vi "EvaluateVariableValues.vi"(8 "error in (no error)":errorcluster, 11 "VariableManager in":refnum<class "VariableManager.lvclass">) -> (0 "error out":errorcluster, 3 "VariableManager out":refnum<class "VariableManager.lvclass">)   [LabVIEW 2013, in "VariableManager.lvclass"]
doc: "Evaluate variable values and store for future acquisition.\n\nAn error is thrown if a sequence function cannot be evaluated."
uses:
  VariableManager.lvclass
  VariableValue/VariableValue.lvclass
  Variable/Variable.lvclass
  PackedLibraries/LuaEvaluatorAPI.lvlibp/API/t_Caching_Expression_Evaluator_Methods_v4.ctl
  SequenceIndex/SequenceIndex.lvclass
  PackedLibraries/LuaEvaluatorAPI.lvlibp
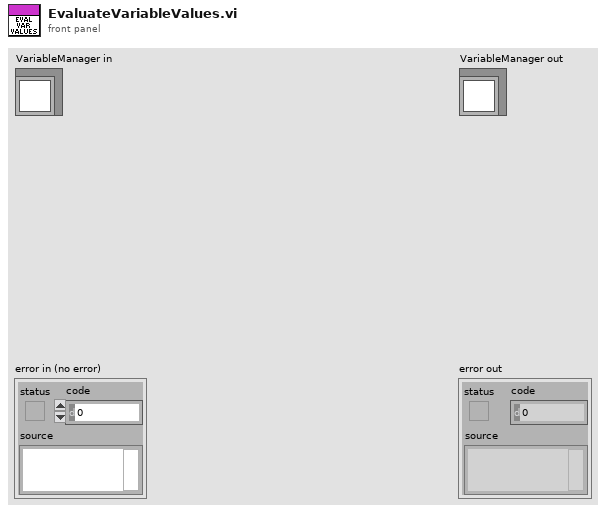
[diagram p1: front panel]
types:
  T1 = typedef "LuaEvaluatorAPI.lvlibp/t_Caching_Expression_Evaluator_Methods_v4.ctl" = enum16{"set", "get", "eval", "eval2", "assign", "execute", "isvalid"}
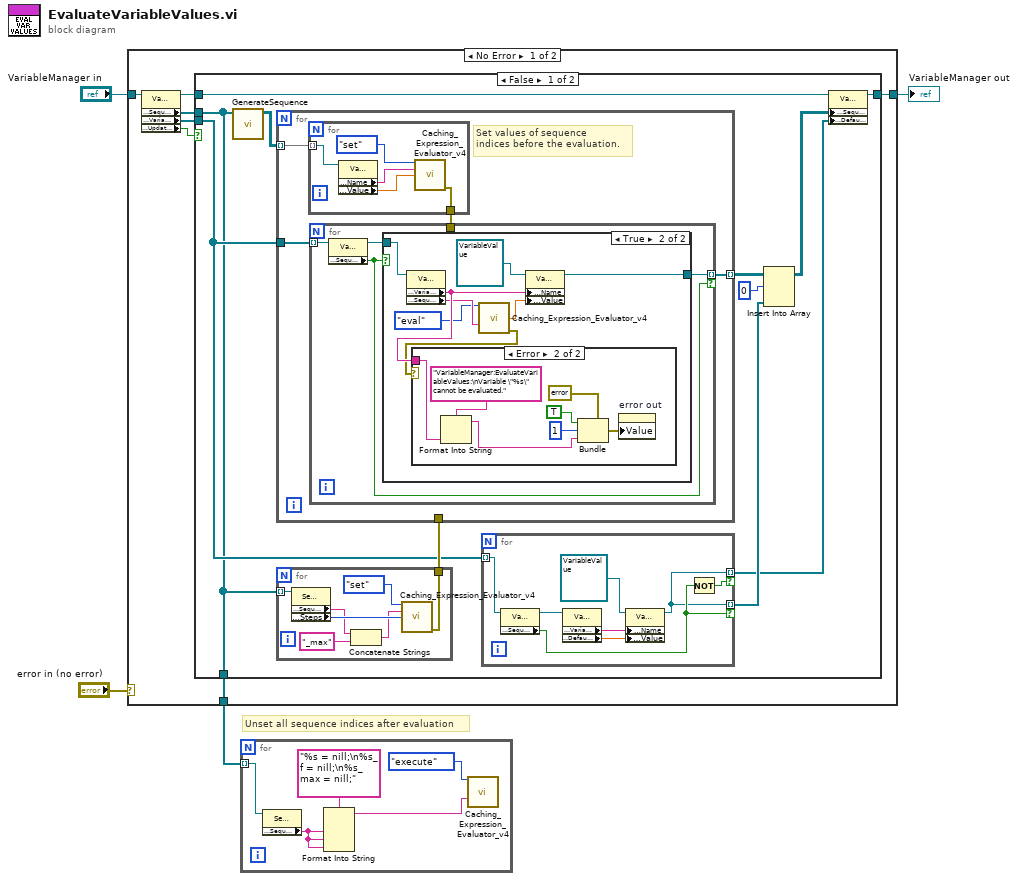
[diagram p0: block diagram]
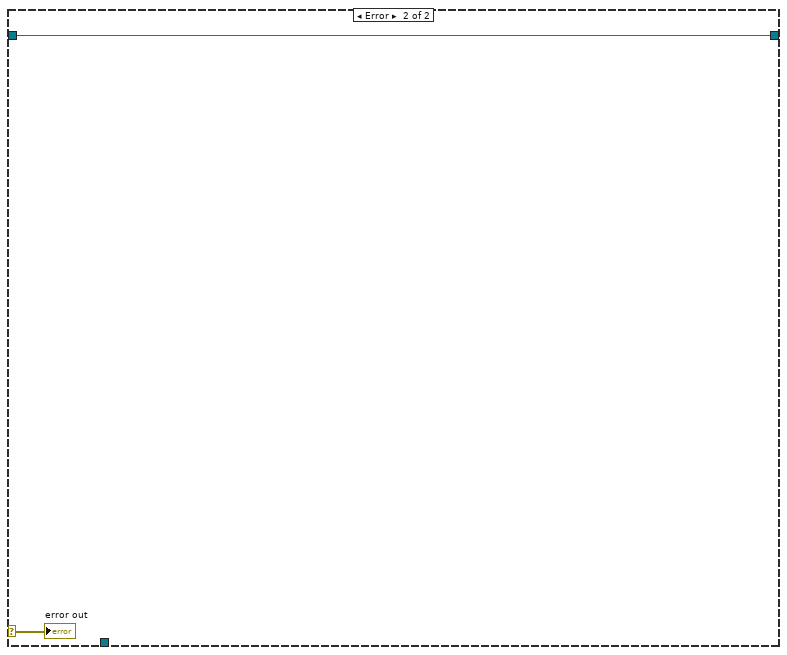
[diagram p5: hidden frame]
diagram:
  # "Unset all sequence indices after evaluation"
  n1 = case shown="No Error" "error in (no error)" {
    selector: "error in (no error)" -> [_ w67]
    tunnel: [w8 w68] -> w3
    tunnel: "VariableManager in" -> [w9 w68]
    tunnel: [w5 _] -> w1
    frame No Error {
      n2 = property class="VariableManager.lvclass"(reference=w9) -> (reference out=w10:refnum<class "VariableManager.lvclass">, "Accessors:SequenceIndices"=w11:refnum<class "SequenceIndex.lvclass">[], "Accessors:Variables"=w7:refnum<class "Variable.lvclass">[], "Accessors:UpdatedValues"=w6:bool)  [unwired: 1 in, 1 out]
      n3 = case shown="False" w6 {
        tunnel: w11 -> [w13 _]
        tunnel: w10 -> [w22 w66]
        tunnel: [w21 w66] -> w8
        tunnel: w7 -> [w14 _]
        tunnel: [w13 _] -> w5
        frame False {
          n4 = call "GenerateSequence.vi"("SequenceIndices"=w13) -> ("SequenceIndexValues"=w12:refnum<class "VariableValue.lvclass">[][])  [unwired: 9 in, 1 out]
          n5 = for {
            tunnel: w13 -> [w29] mode=indexing
            tunnel: [w26] -> w15
            n6 = property class="SequenceIndex.lvclass"(reference=w29) -> ("Accessors:SequenceIndexName"=w24:string, "Accessors:Steps"=w27:u32)  [unwired: 1 in, 2 out]
            n7 = Concatenate Strings(w24, "_max") -> (w23:string)
            n8 = call "Caching_Expression_Evaluator_v4.vi"("method"=t_Caching_Expression_Evaluator_Methods_v4."set", "variable"=w23, "value in"=w27) -> ("error out"=w26:errorcluster)  [unwired: 11 in, 1 out]
          }
          n9 = for {
            tunnel: w12 -> [w41] mode=indexing
            tunnel: w14 -> [w40]
            tunnel: [w39] -> w19 mode=indexing
            tunnel: w15 -> [_]
            # "Set values of sequence \nindices before the evaluation."
            n10 = for {
              tunnel: w41 -> [w65] mode=indexing
              tunnel: [w61] -> w38
              n11 = property class="VariableValue.lvclass"(reference=w65) -> ("Accessors:Name"=w62:string, "Accessors:Value"=w63:dbl)  [unwired: 1 in, 2 out]
              n12 = call "Caching_Expression_Evaluator_v4.vi"("method"=t_Caching_Expression_Evaluator_Methods_v4."set", "variable"=w62, "value in"=w63) -> ("error out"=w61:errorcluster)  [unwired: 11 in, 1 out]
            }
            n13 = for {
              tunnel: w40 -> [w45] mode=indexing
              tunnel: [w43] -> w39 mode=indexing if=w42
              tunnel: w38 -> [_]
              n14 = property class="Variable.lvclass"(reference=w45) -> (reference out=w44:refnum<class "Variable.lvclass">, "Accessors:Sequence"=w42:bool)  [unwired: 1 in, 1 out]
              n15 = case shown="True" w42 {
                tunnel: w44 -> [_ w52]
                tunnel: [_ w51] -> w43
                frame False {
                }
                frame True {
                  n16 = property class="Variable.lvclass"(reference=w52) -> ("Accessors:VariableName"=w50:string, "Accessors:SequenceFunction"=w47:string)  [unwired: 1 in, 2 out]
                  n17 = call "Caching_Expression_Evaluator_v4.vi"("method"=t_Caching_Expression_Evaluator_Methods_v4."eval", "expression/scriptlet"=w47) -> ("value out"=w49:dbl, "error out"=w48:errorcluster)  [unwired: 12 in]
                  n18 = case shown="Error" w48 {
                    tunnel: w50 -> [_ w60]
                    frame No Error {
                    }
                    frame Error {
                      n19 = Format Into String(format string="VariableManager:EvaluateVariableValues:\nVariable \"%s\" cannot be evaluated.", w60) -> (resulting string=w54:string)  [unwired: 2 in, 1 out]
                      n20 = Bundle(cluster=errorcluster {"status"=FALSE, "code"=0, "source"=""} ("error out"), "status"=TRUE, "code"=1, "source"=w54) -> (w57:errorcluster)
                      n21 = property on="error out" class="Clust (strict)"("Value"=w57) -> ()  [unwired: 2 in, 2 out]
                    }
                  }
                  n22 = property class="VariableValue.lvclass"(reference=refnum<class "VariableValue.lvclass"> refnum ("VariableValue.lvclass"), "Accessors:Name"=w50, "Accessors:Value"=w49) -> (reference out=w51:refnum<class "VariableValue.lvclass">)  [unwired: 1 in, 1 out]
                }
              }
            }
          }
          n23 = for {
            tunnel: w14 -> [w37] mode=indexing
            tunnel: [w30] -> w18 mode=indexing if=w35
            tunnel: [w30] -> w16 mode=indexing if=w36
            n24 = property class="Variable.lvclass"(reference=w37) -> (reference out=w32:refnum<class "Variable.lvclass">, "Accessors:Sequence"=w35:bool)  [unwired: 1 in, 1 out]
            n25 = property class="Variable.lvclass"(reference=w32) -> ("Accessors:VariableName"=w34:string, "Accessors:DefaultValue"=w33:dbl)  [unwired: 1 in, 2 out]
            n26 = property class="VariableValue.lvclass"(reference=refnum<class "VariableValue.lvclass"> refnum ("VariableValue.lvclass"), "Accessors:Name"=w34, "Accessors:Value"=w33) -> (reference out=w30:refnum<class "VariableValue.lvclass">)  [unwired: 1 in, 1 out]
            n27 = Not(x=w35) -> (.not. x?=w36:bool)
          }
          n28 = Insert Into Array(array=w19, index (row)=0, new element=w18) -> (w17:refnum<class "VariableValue.lvclass">[][])  [unwired: 1 in]
          n29 = property class="VariableManager.lvclass"(reference=w22, "Accessors:SequenceValues"=w17, "Accessors:DefaultValues"=w16) -> (reference out=w21:refnum<class "VariableManager.lvclass">)  [unwired: 1 in, 1 out]
        }
        frame True {
        }
      }
    }
    frame Error {
      "error out" <- w67
    }
  }
  "VariableManager out" <- w3
  n30 = for {
    tunnel: w1 -> [w72] mode=indexing
    n31 = property class="SequenceIndex.lvclass"(reference=w72) -> ("Accessors:SequenceIndexName"=w71:string)  [unwired: 1 in, 2 out]
    n32 = Format Into String(format string="%s = nill;\n%s_f = nill;\n%s_max = nill;", w71, w71, w71) -> (resulting string=w69:string)  [unwired: 2 in, 1 out]
    n33 = call "Caching_Expression_Evaluator_v4.vi"("method"=t_Caching_Expression_Evaluator_Methods_v4."execute", "expression/scriptlet"=w69) -> ()  [unwired: 12 in, 2 out]
  }
